vi "timekeeper time rate adjustment.vi"(7 "offset":fxp<+/-,19,19>) -> ()   [LabVIEW 2011, in "EPS_Timekeeper.lvlib"]
uses:
  <vilib>/addons/Electrical Power/Example Support/PMU/Time Keeper/EPS_Timekeeper.lvlib
  <vilib>/addons/Electrical Power/Example Support/PMU/Time Keeper/timekeeper time rate adjust valid (g).vi
  <vilib>/addons/Electrical Power/Example Support/PMU/Time Keeper/timekeeper time rate adjust (g).vi
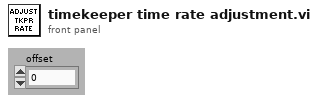
[diagram p1: front panel]
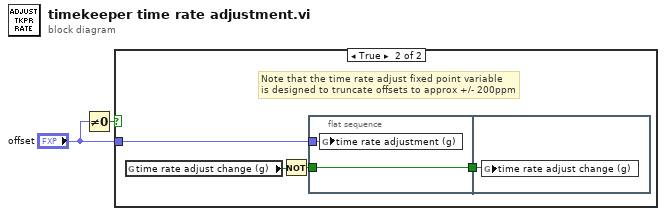
[diagram p0: block diagram]
diagram:
  n1 = Not Equal To 0?(x="offset") -> (x != 0?=w2:bool)
  n2 = case shown="True" w2 {
    tunnel: "offset" -> [_ w3]
    frame False {
    }
    frame True {
      # "Note that the time rate adjust fixed point variable \nis designed to truncate offsets to approx +/- 200ppm"
      n3 = global read "timekeeper time rate adjust valid (g).vi" "time rate adjust change (g)"() -> (w4:bool)
      n4 = Not(x=w4) -> (.not. x?=w5:bool)
      n5 = flat-sequence {
        tunnel: w3 -> [w7]
        tunnel: w5 -> [w8]
        tunnel: [w8] -> w6
        tunnel: w6 -> [w9]
        frame #0 {
          n6 = global write "timekeeper time rate adjust (g).vi" "time rate adjustment (g)"(w7) -> ()
        }
        frame #1 {
          n7 = global write "timekeeper time rate adjust valid (g).vi" "time rate adjust change (g)"(w9) -> ()
        }
      }
    }
  }
